vi "Destroy.vi"(0 "reference":refnum<class "Graph.lvclass">, 5 "error in (no error)":errorcluster) -> (19 "error out":errorcluster)   [LabVIEW 2016, in "Graph.lvclass"]
doc: "Destroys an object created with a Graph constructor VI or a subclass of the Graph class. This VI must be reentrant.\n\n[GOOP 2.1]"
uses:
  <resource>/Framework/Providers/Open_GDS/UML/Graph_class/Graph.lvclass
  <resource>/Framework/Providers/Open_GDS/UML/AbstractEdge_class/AbstractEdge.lvclass
  <resource>/Framework/Providers/Open_GDS/UML/AbstractNode_class/AbstractNode.lvclass
panel:
  out "reference out":refnum<class "Graph.lvclass">
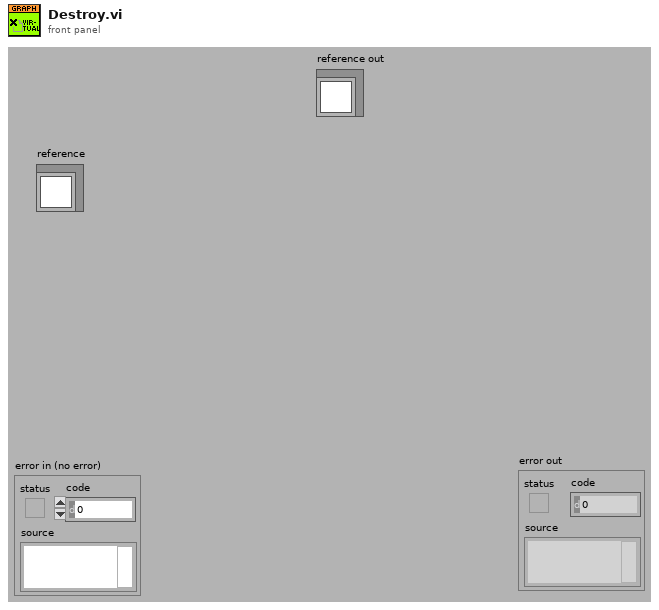
[diagram p1: front panel]
types:
  T1 = typedef "Graph.lvclass/ObjectAttributes.ctl" = cluster{"nodes":refnum<class "AbstractNode.lvclass">[], "edges":refnum<class "AbstractEdge.lvclass">[], "nodesToBeRemoved":refnum<class "AbstractNode.lvclass">[], "edgesToBeRemoved":refnum<class "AbstractEdge.lvclass">[], "needsLayout":bool, "LayoutNodes":refnum<class "AbstractNode.lvclass">[]}
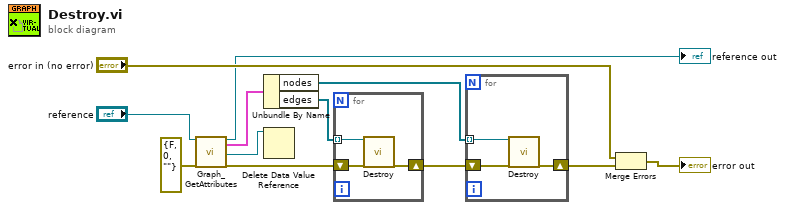
[diagram p0: block diagram]
diagram:
  n1 = call <resource>:"Graph_GetAttributes.vi"("reference in"="reference", "error in (no error)"=errorcluster {"status"=FALSE, "code"=0, "source"=""}) -> ("reference out"=→"reference out":refnum<class "Graph.lvclass">, "Data"=w2:T1, "DataRef"=w1:refnum<data-value>, "error out"=w5:errorcluster)  [unwired: 1 in, 13 out]
  n2 = Unbundle By Name(w2) -> ("nodes"=w6:refnum<class "AbstractNode.lvclass">[], "edges"=w8:refnum<class "AbstractEdge.lvclass">[])
  n3 = Delete Data Value Reference(data value reference=w1) -> ()  [unwired: 1 in, 2 out]
  n4 = for {
    shift-right: [w14] -> w7
    shift-left: w5 -> [w15]
    tunnel: w8 -> [w13] mode=indexing
    n5 = call-dynamic "Destroy.vi"("reference"=w13, "error in (no error)"=w15) -> ("error out"=w14:errorcluster)  [unwired: 17 in]
  }
  n6 = for {
    shift-right: [w17] -> w4
    shift-left: w7 -> [w18]
    tunnel: w6 -> [w16] mode=indexing
    n7 = call-dynamic "Destroy.vi"("reference"=w16, "error in (no error)"=w18) -> ("error out"=w17:errorcluster)  [unwired: 16 in, 1 out]
  }
  n8 = Merge Errors("error in (no error)", w4) -> (→"error out":errorcluster)
